vi "onDestroyHttpSession.vi"(8 "error in (no error)":errorcluster, 11 "http-client in":refnum<class "httpClient.lvclass">) -> (0 "error out":errorcluster, 3 "http-client out":refnum<class "httpClient.lvclass">)   [LabVIEW 2020, in "httpClient.lvlib" / "httpClient.lvclass"]
uses:
  httpClient.lvclass
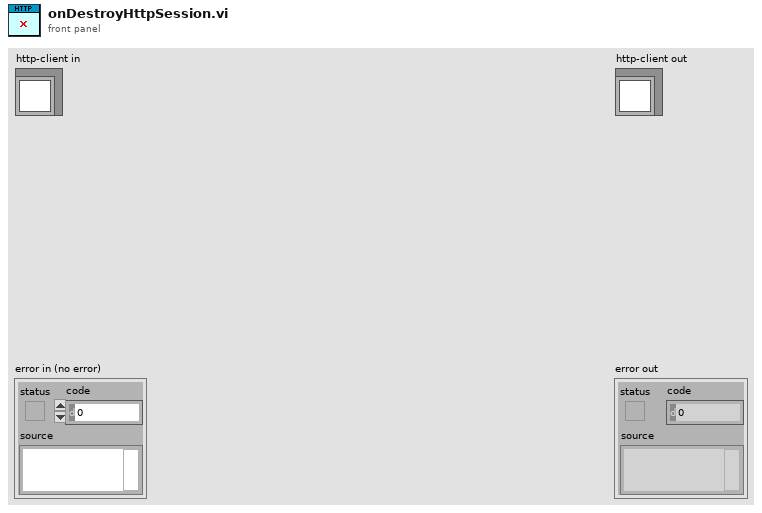
[diagram p1: front panel]
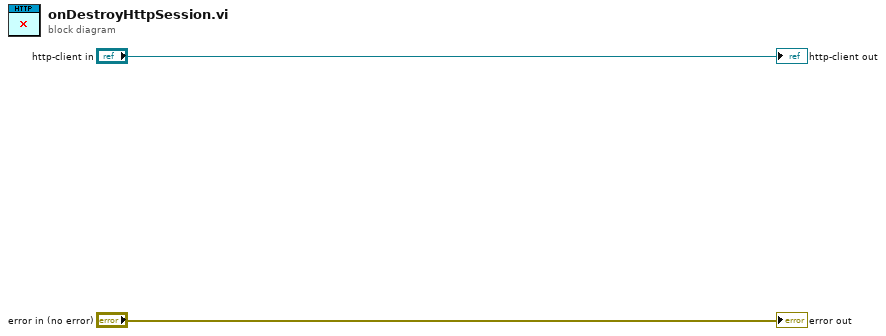
[diagram p0: block diagram]
diagram:
  "error out" <- "error in (no error)"
  "http-client out" <- "http-client in"
